vi "filter.state.vi"(11 "filter.data in":T1 {"memory.command"."order.slot.value"."Quantity" format="%016x"; "memory.command"."order.slot.value"."OrderId" format="%016x"; "memory.command"."ticker.slot.value"."Symbol" format="%016x"; "Scratch"."OrderId" format="%016x"}) -> (3 "filter.data out":T1 {"memory.command"."order.slot.value"."Quantity" format="%016x"; "memory.command"."order.slot.value"."OrderId" format="%016x"; "memory.command"."ticker.slot.value"."Symbol" format="%016x"; "Scratch"."OrderId" format="%016x"})   [LabVIEW 2022 SP3]
uses:
  filter.data.ctl
  filter.states.ctl
  filter.debug.ctl
  filter.debug.slot.ctl
  filter.data.scratch.ctl
  common/orderbook.command.ctl
  common/orderbook.command.type.ctl
  filter.memory.command.ctl
  ticker.slot.ctl
  order.slot.ctl
  filter.getstate.ctl
  filter.getstate.slot.ctl
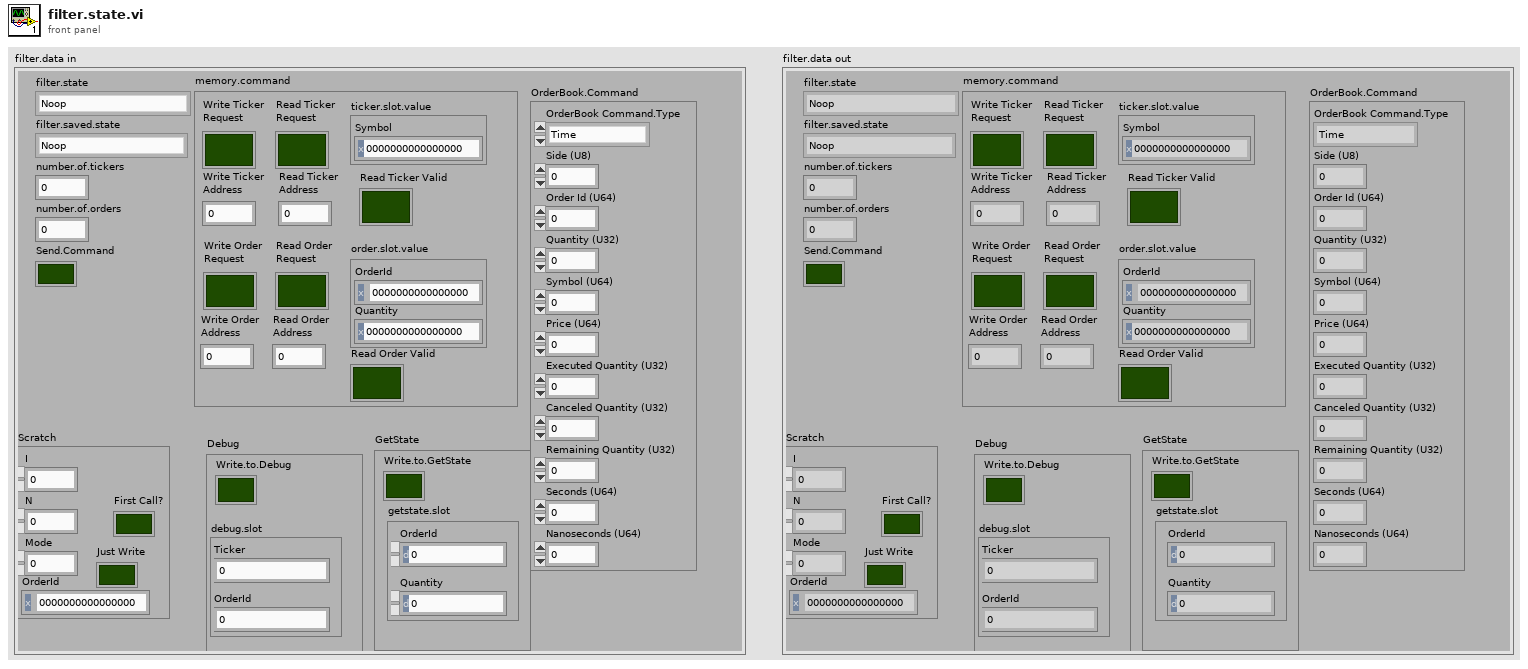
[diagram p1: front panel]
types:
  T1 = typedef "filter.data.ctl" = cluster{"filter.state":T2, "Debug":T3, "number.of.tickers":u32, "number.of.orders":u32, "filter.saved.state":T2, "Scratch":T5, "OrderBook.Command":T6, "Send.Command":bool, "memory.command":T8, "GetState":T11}
  T2 = typedef "filter.states.ctl" = enum16{"Noop", "Reset", "Debug", "Configuration", "Get.State", "Wait.for.Command", "Filter.Add", "Filter.Other", "Insert.Order", "Delete Order"}
  T3 = typedef "filter.debug.ctl" = cluster{"Write.to.Debug":bool, "debug.slot":T4}
  T4 = typedef "filter.debug.slot.ctl" = cluster{"Ticker":u64, "OrderId":u64}
  T5 = typedef "filter.data.scratch.ctl" = cluster{"I":u32, "N":u32, "Mode":u32, "OrderId":u64, "First Call?":bool, "Just Write":bool}
  T6 = typedef "orderbook.command.ctl" = cluster{"OrderBook Command.Type":T7, "Side (U8)":u8, "Order Id (U64)":u64, "Quantity (U32)":u32, "Symbol (U64)":u64, "Price (U64)":u64, "Executed Quantity (U32)":u32, "Canceled Quantity (U32)":u32, "Remaining Quantity (U32)":u32, "Seconds (U64)":u64, "Nanoseconds (U64)":u64}
  T7 = typedef "orderbook.command.type.ctl" = enum16{"Time", "AddOrder", "OrderExecuted", "OrderExecutedAtPrice", "ReduceSize", "ModifyOrder", "DeleteOrder", "Get.State", "Get.All.Orders", "Get.Top"}
  T8 = typedef "filter.memory.command.ctl" = cluster{"ticker.slot.value":T9, "order.slot.value":T10, "Write Ticker\nAddress":u32, "Write Ticker\nRequest":bool, "Read Ticker\nRequest":bool, "Read Ticker\nAddress":u32, "Read Ticker Valid":bool, "Write Order\nAddress":u32, "Write Order\nRequest":bool, "Read Order\nRequest":bool, "Read Order\nAddress":u32, "Read Order Valid":bool}
  T9 = typedef "ticker.slot.ctl" = cluster{"Symbol":u64}
  T10 = typedef "order.slot.ctl" = cluster{"OrderId":u64, "Quantity":u64}
  T11 = typedef "filter.getstate.ctl" = cluster{"Write.to.GetState":bool, "getstate.slot":T12}
  T12 = typedef "filter.getstate.slot.ctl" = cluster{"OrderId":u64, "Quantity":u64}
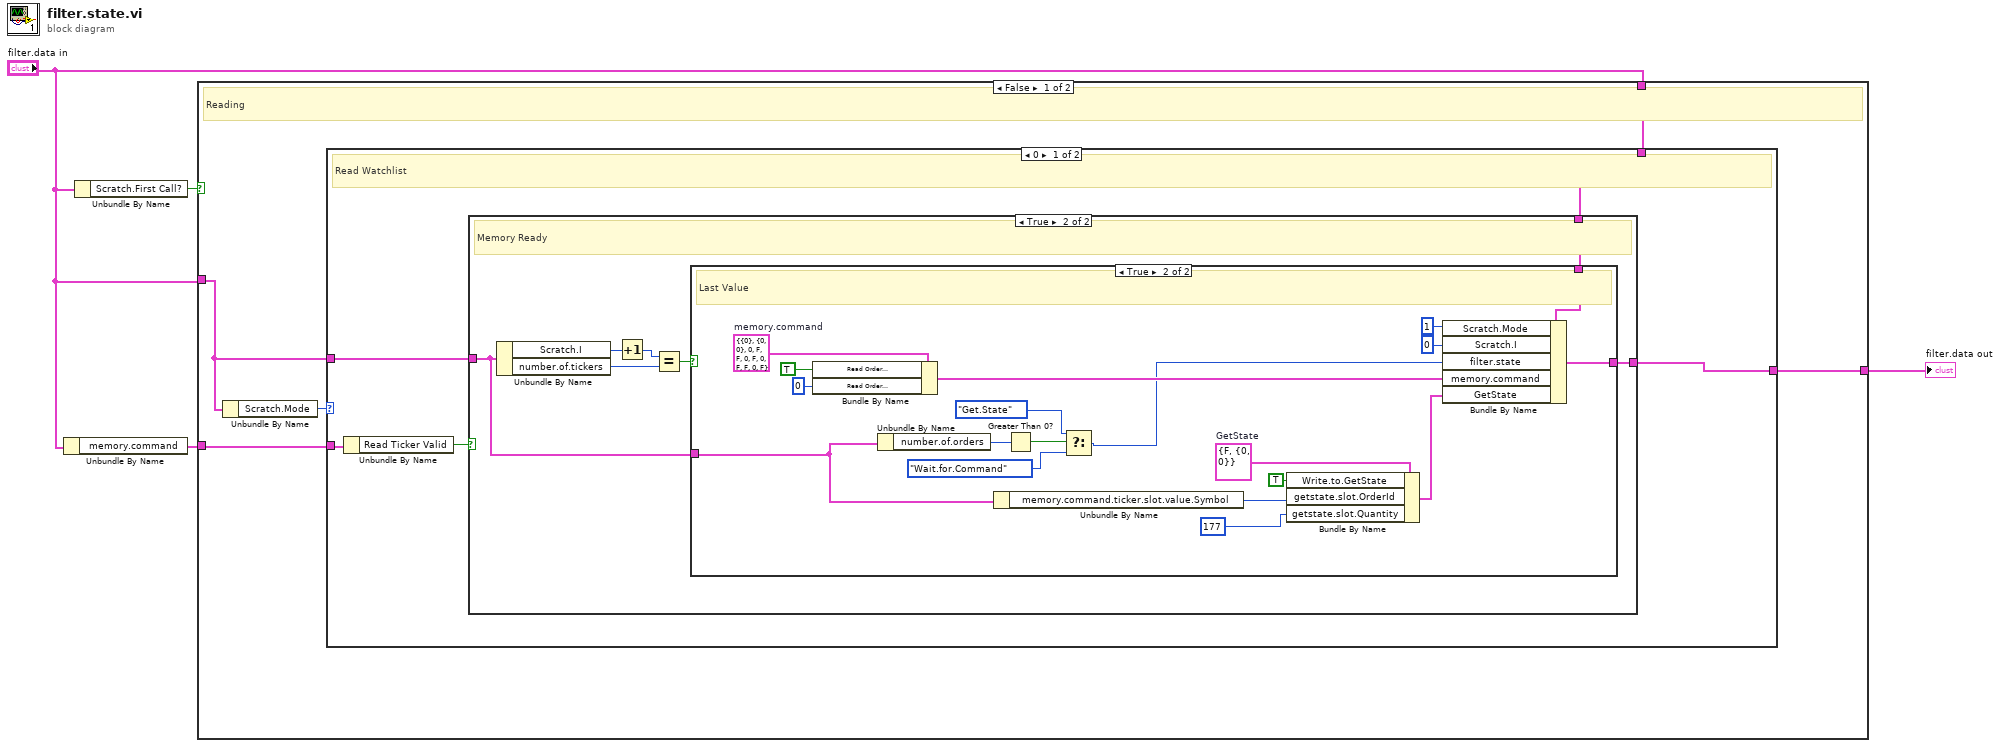
[diagram p0: block diagram]
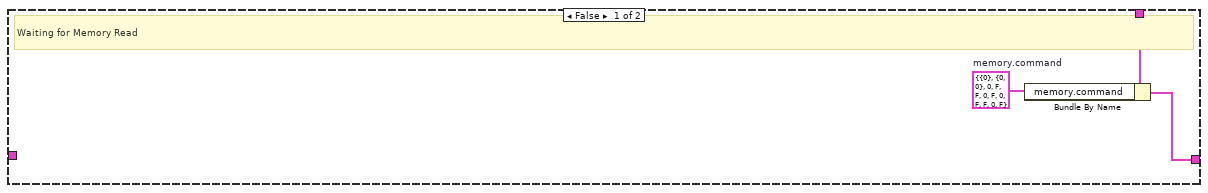
[diagram p2: hidden frame]
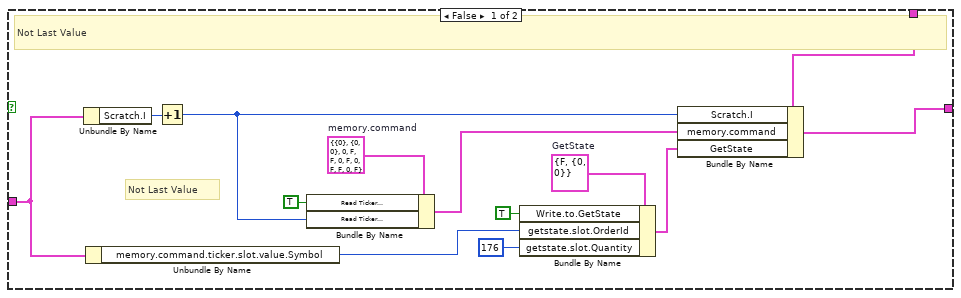
[diagram p3: hidden frame]
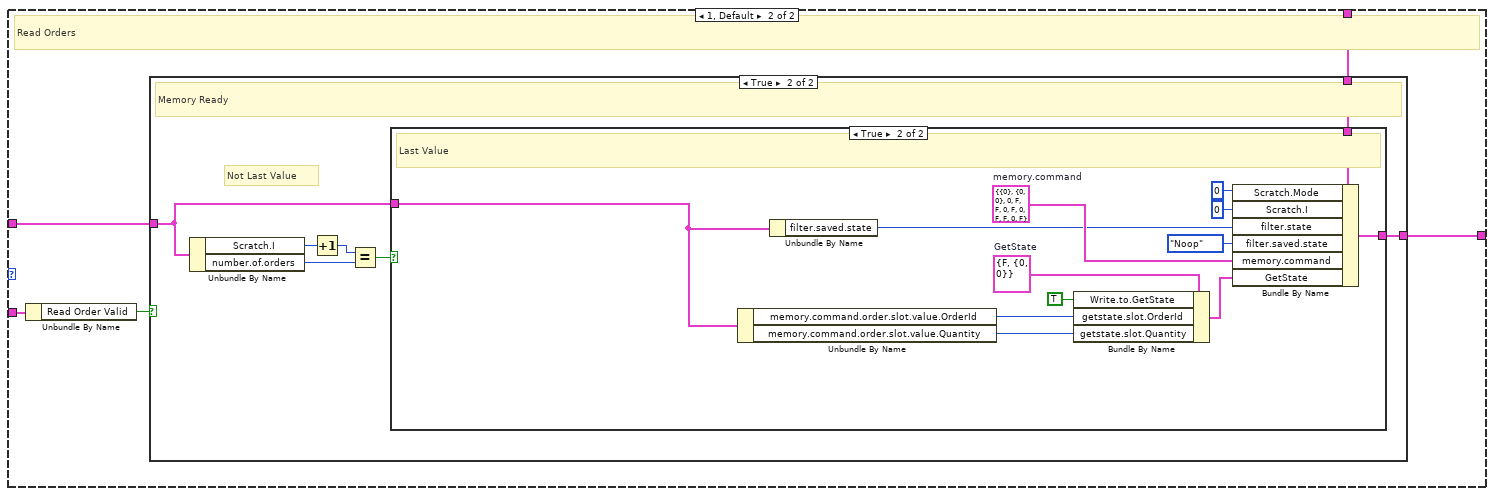
[diagram p4: hidden frame]
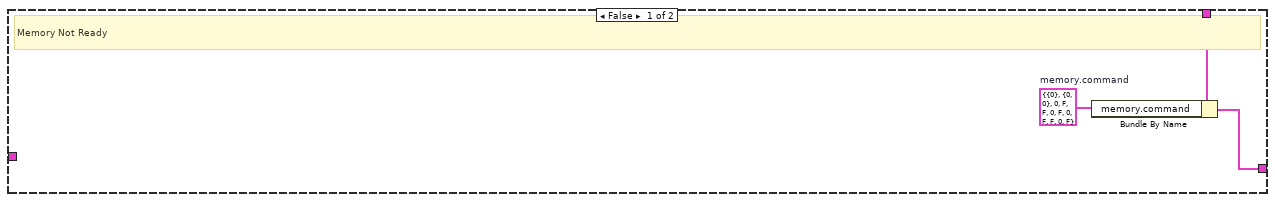
[diagram p5: hidden frame]
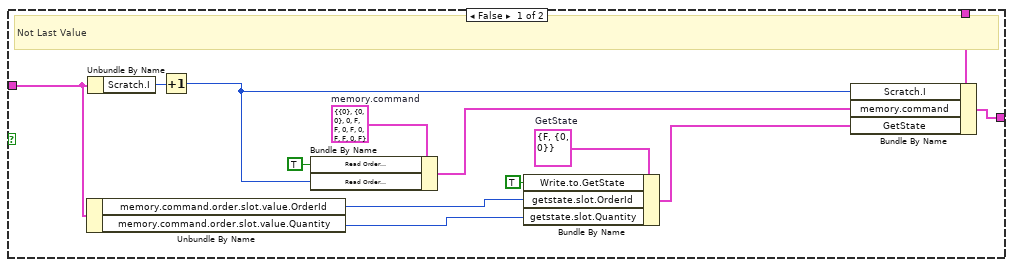
[diagram p6: hidden frame]
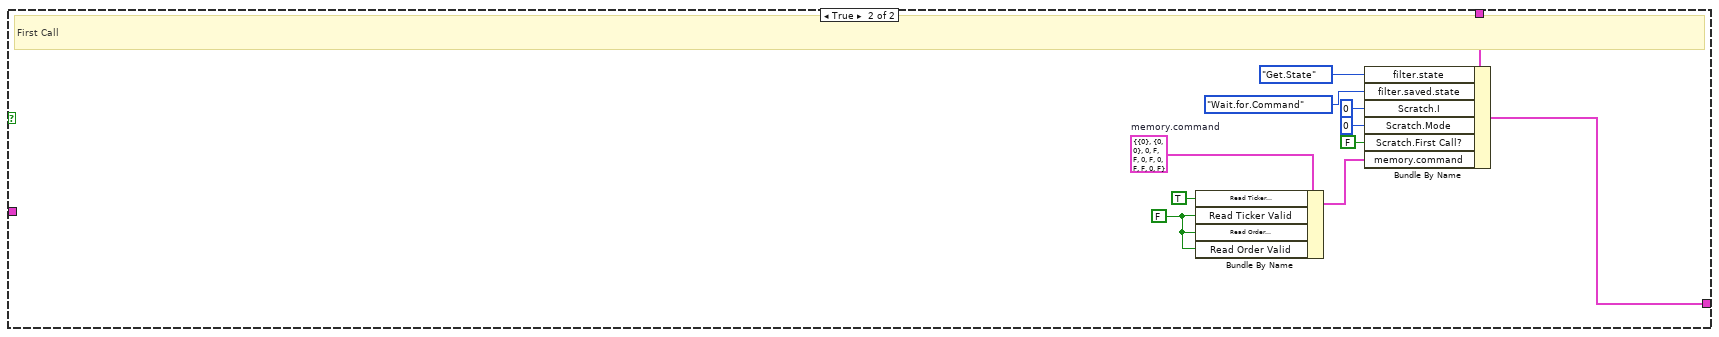
[diagram p7: hidden frame]
diagram:
  n1 = Unbundle By Name("filter.data in") -> ("memory.command"=w4:T8)
  n2 = Unbundle By Name("filter.data in") -> ("Scratch.First Call?"=w1:bool)
  n3 = case shown="False" w1 {
    tunnel: "filter.data in" -> [w8 w108]
    tunnel: [w9 w107] -> w2
    tunnel: "filter.data in" -> [w6 _]
    tunnel: w4 -> [w7 _]
    frame False {
      # "Reading"
      n4 = Unbundle By Name(w6) -> ("Scratch.Mode"=w5:u32)
      n5 = case shown="0" w5 {
        tunnel: [w14 w61] -> w9
        tunnel: w8 -> [w13 w60]
        tunnel: w7 -> [w11 w58]
        tunnel: w6 -> [w10 w57]
        frame 0 {
          # "Read Watchlist"
          n6 = Unbundle By Name(w11) -> ("Read Ticker Valid"=w12:bool)
          n7 = case shown="True" w12 {
            tunnel: [w15 w18] -> w14
            tunnel: w13 -> [w17 w19]
            tunnel: w10 -> [_ w20]
            frame False {
              w16 = T8 {"ticker.slot.value"={"Symbol"=0}, "order.slot.value"={"OrderId"=0, "Quantity"=0}, "Write Ticker\nAddress"=0, "Write Ticker\nRequest"=FALSE, "Read Ticker\nRequest"=FALSE, "Read Ticker\nAddress"=0, "Read Ticker Valid"=FALSE, "Write Order\nAddress"=0, "Write Order\nRequest"=FALSE, "Read Order\nRequest"=FALSE, "Read Order\nAddress"=0, "Read Order Valid"=FALSE}  # memory.command
              # "Waiting for Memory Read"
              n8 = Bundle By Name(cluster=w17, "memory.command"=w16) -> (w15:T1)
            }
            frame True {
              # "Memory Ready"
              n9 = Unbundle By Name(w20) -> ("Scratch.I"=w24:u32, "number.of.tickers"=w22:u32)
              n10 = Increment(x=w24) -> (x+1=w23:u32)
              n11 = Equal?(x=w23, y=w22) -> (x = y?=w21:bool)
              n12 = case shown="True" w21 {
                tunnel: w20 -> [w30 w43]
                tunnel: w19 -> [w26 w56]
                tunnel: [w37 w55] -> w18
                frame False {
                  w33 = T11 {"Write.to.GetState"=FALSE, "getstate.slot"={"OrderId"=0, "Quantity"=0}}  # GetState
                  w36 = T8 {"ticker.slot.value"={"Symbol"=0}, "order.slot.value"={"OrderId"=0, "Quantity"=0}, "Write Ticker\nAddress"=0, "Write Ticker\nRequest"=FALSE, "Read Ticker\nRequest"=FALSE, "Read Ticker\nAddress"=0, "Read Ticker Valid"=FALSE, "Write Order\nAddress"=0, "Write Order\nRequest"=FALSE, "Read Order\nRequest"=FALSE, "Read Order\nAddress"=0, "Read Order Valid"=FALSE}  # memory.command
                  # "Not Last Value"
                  # "Not Last Value"
                  n13 = Unbundle By Name(w30) -> ("Scratch.I"=w34:u32)
                  n14 = Unbundle By Name(w30) -> ("memory.command.ticker.slot.value.Symbol"=w29:u64)
                  n15 = Increment(x=w34) -> (x+1=w27:u32)
                  n16 = Bundle By Name(cluster=w36, "Read Ticker\nRequest"=TRUE ("Read.Request"), "Read Ticker\nAddress"=w27) -> (w35:T8)
                  n17 = Bundle By Name(cluster=w33, "Write.to.GetState"=TRUE ("Write.to.Debug"), "getstate.slot.OrderId"=w29, "getstate.slot.Quantity"=u64 176 ("debug.slot.OrderId")) -> (w32:T11)
                  n18 = Bundle By Name(cluster=w26, "Scratch.I"=w27, "memory.command"=w35, "GetState"=w32) -> (w37:T1)
                }
                frame True {
                  w44 = T11 {"Write.to.GetState"=FALSE, "getstate.slot"={"OrderId"=0, "Quantity"=0}}  # GetState
                  w48 = T8 {"ticker.slot.value"={"Symbol"=0}, "order.slot.value"={"OrderId"=0, "Quantity"=0}, "Write Ticker\nAddress"=0, "Write Ticker\nRequest"=FALSE, "Read Ticker\nRequest"=FALSE, "Read Ticker\nAddress"=0, "Read Ticker Valid"=FALSE, "Write Order\nAddress"=0, "Write Order\nRequest"=FALSE, "Read Order\nRequest"=FALSE, "Read Order\nAddress"=0, "Read Order Valid"=FALSE}  # memory.command
                  # "Last Value"
                  n19 = Bundle By Name(cluster=w48, "Read Order\nRequest"=TRUE ("Read Order\nRequest"), "Read Order\nAddress"=u32 0 ("Read Order\nAddress")) -> (w47:T8)
                  n20 = Unbundle By Name(w43) -> ("number.of.orders"=w42:u32)
                  n21 = Unbundle By Name(w43) -> ("memory.command.ticker.slot.value.Symbol"=w52:u64)
                  n22 = Greater Than 0?(x=w42) -> (x > 0?=w41:bool)
                  n23 = Select(t=filter.states."Get.State" ("filter.state"), s=w41, f=filter.states."Wait.for.Command") -> (s? t:f=w39:T2)
                  n24 = Bundle By Name(cluster=w44, "Write.to.GetState"=TRUE ("Write.to.Debug"), "getstate.slot.OrderId"=w52, "getstate.slot.Quantity"=u64 177 ("debug.slot.OrderId")) -> (w54:T11)
                  n25 = Bundle By Name(cluster=w56, "Scratch.Mode"=u32 1, "Scratch.I"=u32 0, "filter.state"=w39, "memory.command"=w47, "GetState"=w54) -> (w55:T1)
                }
              }
            }
          }
        }
        frame 1, Default {
          # "Read Orders"
          n26 = Unbundle By Name(w58) -> ("Read Order Valid"=w59:bool)
          n27 = case shown="True" w59 {
            tunnel: [w62 w65] -> w61
            tunnel: w60 -> [w64 w66]
            tunnel: w57 -> [_ w67]
            frame False {
              w63 = T8 {"ticker.slot.value"={"Symbol"=0}, "order.slot.value"={"OrderId"=0, "Quantity"=0}, "Write Ticker\nAddress"=0, "Write Ticker\nRequest"=FALSE, "Read Ticker\nRequest"=FALSE, "Read Ticker\nAddress"=0, "Read Ticker Valid"=FALSE, "Write Order\nAddress"=0, "Write Order\nRequest"=FALSE, "Read Order\nRequest"=FALSE, "Read Order\nAddress"=0, "Read Order Valid"=FALSE}  # memory.command
              # "Memory Not Ready"
              n28 = Bundle By Name(cluster=w64, "memory.command"=w63) -> (w62:T1)
            }
            frame True {
              # "Not Last Value"
              # "Memory Ready"
              n29 = Unbundle By Name(w67) -> ("Scratch.I"=w71:u32, "number.of.orders"=w69:u32)
              n30 = Increment(x=w71) -> (x+1=w70:u32)
              n31 = Equal?(x=w70, y=w69) -> (x = y?=w68:bool)
              n32 = case shown="True" w68 {
                tunnel: w67 -> [w78 w93]
                tunnel: w66 -> [w76 w97]
                tunnel: [w84 w96] -> w65
                frame False {
                  w72 = T11 {"Write.to.GetState"=FALSE, "getstate.slot"={"OrderId"=0, "Quantity"=0}}  # GetState
                  w83 = T8 {"ticker.slot.value"={"Symbol"=0}, "order.slot.value"={"OrderId"=0, "Quantity"=0}, "Write Ticker\nAddress"=0, "Write Ticker\nRequest"=FALSE, "Read Ticker\nRequest"=FALSE, "Read Ticker\nAddress"=0, "Read Ticker Valid"=FALSE, "Write Order\nAddress"=0, "Write Order\nRequest"=FALSE, "Read Order\nRequest"=FALSE, "Read Order\nAddress"=0, "Read Order Valid"=FALSE}  # memory.command
                  # "Not Last Value"
                  n33 = Unbundle By Name(w78) -> ("memory.command.order.slot.value.OrderId"=w73:u64, "memory.command.order.slot.value.Quantity"=w74:u64)
                  n34 = Unbundle By Name(w78) -> ("Scratch.I"=w81:u32)
                  n35 = Increment(x=w81) -> (x+1=w75:u32)
                  n36 = Bundle By Name(cluster=w83, "Read Order\nRequest"=TRUE ("Read.Request"), "Read Order\nAddress"=w75) -> (w82:T8)
                  n37 = Bundle By Name(cluster=w72, "Write.to.GetState"=TRUE ("Write.to.Debug"), "getstate.slot.OrderId"=w73, "getstate.slot.Quantity"=w74) -> (w80:T11)
                  n38 = Bundle By Name(cluster=w76, "Scratch.I"=w75, "memory.command"=w82, "GetState"=w80) -> (w84:T1)
                }
                frame True {
                  w85 = T11 {"Write.to.GetState"=FALSE, "getstate.slot"={"OrderId"=0, "Quantity"=0}}  # GetState
                  w92 = T8 {"ticker.slot.value"={"Symbol"=0}, "order.slot.value"={"OrderId"=0, "Quantity"=0}, "Write Ticker\nAddress"=0, "Write Ticker\nRequest"=FALSE, "Read Ticker\nRequest"=FALSE, "Read Ticker\nAddress"=0, "Read Ticker Valid"=FALSE, "Write Order\nAddress"=0, "Write Order\nRequest"=FALSE, "Read Order\nRequest"=FALSE, "Read Order\nAddress"=0, "Read Order Valid"=FALSE}  # memory.command
                  # "Last Value"
                  n39 = Unbundle By Name(w93) -> ("memory.command.order.slot.value.OrderId"=w87:u64, "memory.command.order.slot.value.Quantity"=w86:u64)
                  n40 = Unbundle By Name(w93) -> ("filter.saved.state"=w91:T2)
                  n41 = Bundle By Name(cluster=w85, "Write.to.GetState"=TRUE ("Write.to.Debug"), "getstate.slot.OrderId"=w87, "getstate.slot.Quantity"=w86) -> (w95:T11)
                  n42 = Bundle By Name(cluster=w97, "Scratch.Mode"=u32 0, "Scratch.I"=u32 0, "filter.state"=w91, "filter.saved.state"=filter.states."Noop", "memory.command"=w92, "GetState"=w95) -> (w96:T1)
                }
              }
            }
          }
        }
      }
    }
    frame True {
      w101 = FALSE ("Read Ticker Valid")
      w103 = T8 {"ticker.slot.value"={"Symbol"=0}, "order.slot.value"={"OrderId"=0, "Quantity"=0}, "Write Ticker\nAddress"=0, "Write Ticker\nRequest"=FALSE, "Read Ticker\nRequest"=FALSE, "Read Ticker\nAddress"=0, "Read Ticker Valid"=FALSE, "Write Order\nAddress"=0, "Write Order\nRequest"=FALSE, "Read Order\nRequest"=FALSE, "Read Order\nAddress"=0, "Read Order Valid"=FALSE}  # memory.command
      # "First Call"
      n43 = Bundle By Name(cluster=w103, "Read Ticker\nRequest"=TRUE ("Read Ticker\nRequest"), "Read Ticker Valid"=w101, "Read Order\nRequest"=w101, "Read Order Valid"=w101) -> (w99:T8)
      n44 = Bundle By Name(cluster=w108, "filter.state"=filter.states."Get.State", "filter.saved.state"=filter.states."Wait.for.Command", "Scratch.I"=u32 0, "Scratch.Mode"=u32 0, "Scratch.First Call?"=FALSE, "memory.command"=w99) -> (w107:T1)
    }
  }
  "filter.data out" <- w2
